vi "Test Serialize Variants.vi"(8 "error in (no error)":errorcluster) -> (0 "error out":errorcluster)   [LabVIEW 2013]
uses:
  src/Serializer/JSON Serializer/JSON Serializer.lvclass
  <vilib>/addons/_JKI Toolkits/Caraya/classes/Test/Test.lvclass
  <vilib>/addons/_JKI Toolkits/Caraya/classes/Assert/Assert.lvclass
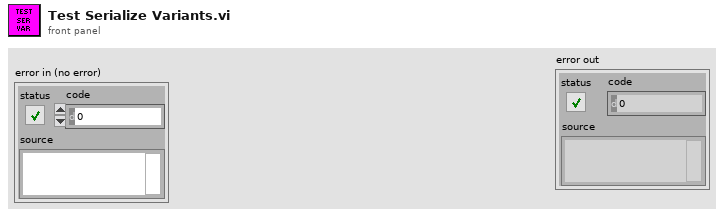
[diagram p1: front panel]
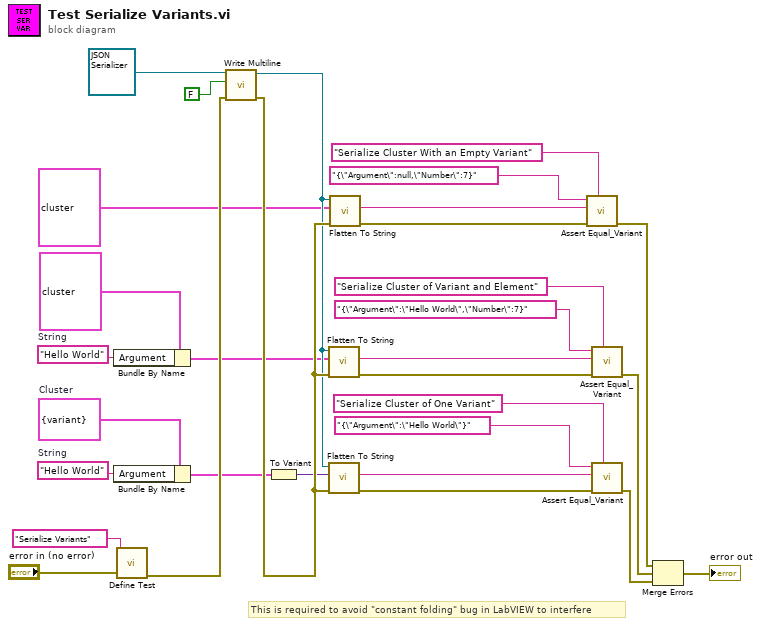
[diagram p0: block diagram]
diagram:
  w12 = "Hello World"  # String
  w11 = cluster{"Argument":variant} {"Argument"=variant}  # Cluster
  w14 = "Hello World"  # String
  # "This is required to avoid \"constant folding\" bug in LabVIEW to interfere"
  n1 = Bundle By Name(cluster=cluster{"Argument":variant, "Number":i32} {"Argument"=variant, "Number"=7}, "Argument"=w14) -> (w13:cluster{"Argument":variant, "Number":i32})
  n2 = Bundle By Name(cluster=w11, "Argument"=w12) -> (w6:cluster{"Argument":variant})
  n3 = call <vilib>:"Define Test.vi"("error in (no error)"="error in (no error)", "Label (VI Title)"="Serialize Variants") -> ("error out"=w26:errorcluster)  [unwired: 9 in]
  n4 = call-dynamic "Write Multiline.vi"("error in (no error)"=w26, "Multiline"=FALSE, "JSON Serializer in"=refnum<class "JSON Serializer.lvclass"> refnum ("JKI JSON Serialization.lvlib:JSON Serializer.lvclass")) -> ("error out"=w23:errorcluster, "JSON Serializer out"=w22:refnum<class "JSON Serializer.lvclass">)  [unwired: 7 in]
  n5 = To Variant(anything=w6) -> (Variant=w5:variant)
  n6 = call-dynamic "Flatten To String.vi"("error in (no error)"=w23, "Variant"=w13, "JSON Serializer in"=w22) -> ("error out"=w4:errorcluster, "String"=w3:string)  [unwired: 6 in, 1 out]
  n7 = call-dynamic "Flatten To String.vi"("error in (no error)"=w23, "Variant"=w5, "JSON Serializer in"=w22) -> ("error out"=w8:errorcluster, "String"=w7:string)  [unwired: 6 in, 1 out]
  n8 = call-dynamic "Flatten To String.vi"("error in (no error)"=w23, "Variant"=cluster{"Argument":variant, "Number":i32} {"Argument"=variant, "Number"=7}, "JSON Serializer in"=w22) -> ("error out"=w20:errorcluster, "String"=w17:string)  [unwired: 6 in, 1 out]
  n9 = call <vilib>:"Assert Equal_Variant.vi"("Label"="Serialize Cluster With an Empty Variant", "error in (no error)"=w20, "Y"=w17, "X"="{\"Argument\":null,\"Number\":7}") -> ("error out"=w16:errorcluster)  [unwired: 7 in]
  n10 = call <vilib>:"Assert Equal_Variant.vi"("Label"="Serialize Cluster of Variant and Element", "error in (no error)"=w4, "Y"=w3, "X"="{\"Argument\":\"Hello World\",\"Number\":7}") -> ("error out"=w29:errorcluster)  [unwired: 7 in]
  n11 = call <vilib>:"Assert Equal_Variant.vi"("Label"="Serialize Cluster of One Variant", "error in (no error)"=w8, "Y"=w7, "X"="{\"Argument\":\"Hello World\"}") -> ("error out"=w24:errorcluster)  [unwired: 7 in]
  n12 = Merge Errors(w16, w29, w24) -> (→"error out":errorcluster)
